vi "PIDControllers.vi"() -> ()   [LabVIEW 2018]
uses:
  <vilib>/Platform/TimedLoop/XDataNode/timing_clust.ctl
  <vilib>/Platform/TimedLoop/XDataNode/nitl_modes.ctl
  <vilib>/Platform/TimedLoop/XDataNode/wakeup.ctl
  Modbus/ControllersHost/BPCS Global Variables.vi
  <vilib>/addons/control/pid/pid.llb/PID Advanced (DBL).vi
  <vilib>/Platform/TimedLoop/XDataNode/XDataNode.xnode
  <vilib>/Platform/TimedLoop/XDataNode/XDNodeRunTimeDep.lvlib
  <vilib>/addons/control/pid/NI_PID_pid.lvlib
panel:
  in  "stop":bool
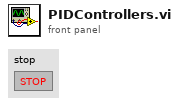
[diagram p1: front panel]
types:
  T1 = typedef "XDNodeRunTimeDep.lvlib/timing_clust.ctl" = cluster{"Expected End [f-1]":u64, "Actual End [f-1]":u64, "Finished Late? [f-1]":bool, "Expected End [i-1]":u64, "Actual End [i-1]":u64, "Finished Late? [i-1]":bool, "Expected Start [i]":u64, "Actual Start [i]":u64, "Expected Start [f]":u64, "Actual Start [f]":u64, "Source Name":string, "Structure Name":string, "Period":i64, "Deadline":i64, "Offset":i64, "Start":i64, "Priority":i32, "Timeout":i32, "Mode":T2, "Wakeup Reason":T3, "Error":errorcluster, "Source Type":string, "Secondary Source Type":string, "Global End Time":u64, "Global Start Time":u64, "Frame Duration":u64, "Iteration Duration":u64, "Assigned CPU":i32, "I/O Scan Engine Mode":u32}
  T2 = typedef "XDNodeRunTimeDep.lvlib/nitl_modes.ctl" = enum32{"No Change", "Process missed periods, maintain original phase", "Discard missed periods, maintain original phase", "Process missed periods, ignore original phase", "Discard missed periods, ignore original phase"}
  T3 = typedef "XDNodeRunTimeDep.lvlib/wakeup.ctl" = enum32{"Normal", "Aborted", "Asynchronous wakeup", "Timing source error", "Timed loop error", "Timeout"}
  T4 = cluster{"HMI-10LIC200-KPID[0]":dbl, "HMI-10LIC200-KPID[1]":dbl, "HMI-10LIC200-KPID[2]":dbl}
  T5 = cluster{"HMI-10TIC100-KPID[0]":dbl, "HMI-10TIC100-KPID[1]":dbl, "HMI-10TIC100-KPID[2]":dbl}
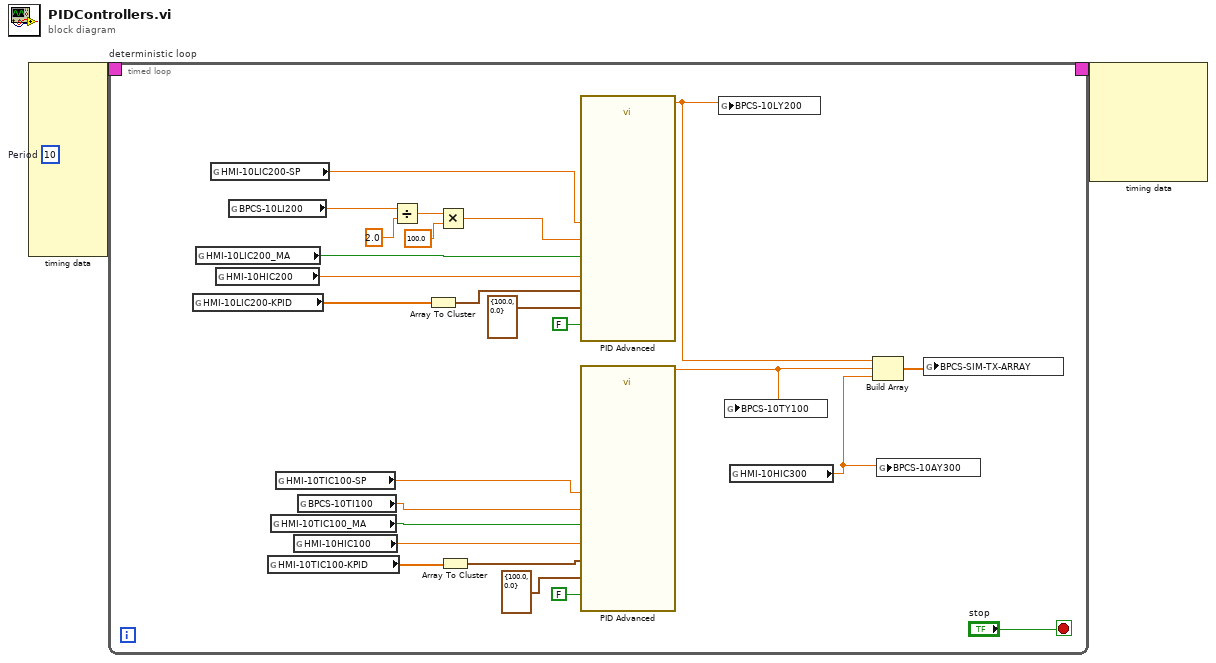
[diagram p0: block diagram]
diagram:
  w1 = i64 10  # Period
  n1 = node-c288 ("Input Node")(w1) -> (w3:T1)  [unwired: 9 in]
  n2 = timed-loop "deterministic loop" {
    timing: w3 -> [_]
    timing-out: [_] -> w2
    stop <- "stop" stop-if-true
    n3 = global read "BPCS Global Variables.vi" "HMI-10LIC200-KPID"() -> (w9:dbl[])
    n4 = global read "BPCS Global Variables.vi" "HMI-10LIC200_MA"() -> (w5:bool)
    n5 = global read "BPCS Global Variables.vi" "HMI-10LIC200-SP"() -> (w11:dbl)
    n6 = global read "BPCS Global Variables.vi" "HMI-10HIC200"() -> (w10:dbl)
    n7 = global read "BPCS Global Variables.vi" "BPCS-10LI200"() -> (w17:dbl)
    n8 = global read "BPCS Global Variables.vi" "HMI-10TIC100-KPID"() -> (w6:dbl[])
    n9 = global read "BPCS Global Variables.vi" "HMI-10TIC100_MA"() -> (w4:bool)
    n10 = global read "BPCS Global Variables.vi" "HMI-10TIC100-SP"() -> (w8:dbl)
    n11 = global read "BPCS Global Variables.vi" "HMI-10HIC100"() -> (w7:dbl)
    n12 = global read "BPCS Global Variables.vi" "BPCS-10TI100"() -> (w16:dbl)
    n13 = Divide(x=w17, y=2.0 ("x")) -> (x/y=w27:dbl)
    n14 = Array To Cluster(array=w9) -> (cluster=w24:T4)
    n15 = Multiply(x=w27, y=100.0) -> (x*y=w25:dbl)
    n16 = Array To Cluster(array=w6) -> (cluster=w21:T5)
    n17 = call-poly <vilib>:"PID Advanced.vi"("setpoint"=w11, "output range"=cluster{"output high":dbl, "output low":dbl} {"output high"=100.0, "output low"=0.0}, "auto? (T)"=w5, "manual control"=w10, "process variable"=w25, "PID gains"=w24, "reinitialize? (F)"=FALSE) -> ("output"=w15:dbl)  [unwired: 7 in, 1 out]
    n18 = call-poly <vilib>:"PID Advanced.vi"("setpoint"=w8, "output range"=cluster{"output high":dbl, "output low":dbl} {"output high"=100.0, "output low"=0.0}, "auto? (T)"=w4, "manual control"=w7, "process variable"=w16, "PID gains"=w21, "reinitialize? (F)"=FALSE) -> ("output"=w14:dbl)  [unwired: 7 in, 1 out]
    n19 = global write "BPCS Global Variables.vi" "BPCS-10LY200"(w15) -> ()
    n20 = global write "BPCS Global Variables.vi" "BPCS-10TY100"(w14) -> ()
    n21 = global read "BPCS Global Variables.vi" "HMI-10HIC300"() -> (w12:dbl)
    n22 = Build Array(w15, w14, w12) -> (w13:dbl[])
    n23 = global write "BPCS Global Variables.vi" "BPCS-10AY300"(w12) -> ()
    n24 = global write "BPCS Global Variables.vi" "BPCS-SIM-TX-ARRAY"(w13) -> ()
  }
  n25 = node-c288 ("Output Node")(w2) -> ()  [unwired: 6 out]
